vi "TSM SSC DCPower Finish Waveform Acquisition.vi"(0 "DCPower SSC in":T3, 1 "Settings":T1 {"Previous Settings"."Triggers:Measure Trigger:Trigger Type" items=["Digital Edge"=1014, "Software Edge"=1015, "None"=1012]; "Previous Settings"."Measurement:Advanced:Measure When" items=["Automatically after Source Complete"=1025, "On Demand"=1026, "On Measure Trigger"=1027]; "Previous Settings"."Measurement:Aperture Time" format="%#_6p"; "Previous Settings"."Measurement:Aperture Time Units" items=["Seconds"=1028, "Power Line Cycles"=1029]}, 5 "Fetch Waveform Length (s)":dbl, 11 "error in":errorcluster) -> (4 "DCPower SSC out":T3, 6 "Voltage Waveforms":waveform(dbl)[](graph), 8 "Current Waveforms":waveform(dbl)[](graph), 15 "error out":errorcluster)   [LabVIEW 2019]
doc: "This VI reconfigures the SMU to the previous settings and outputs the samples captured during waveform acquisition."
uses:
  TSM/TSM SSC DCPower.ctl
  <vilib>/NI_TestStand_SemiconductorModule/NI_TestStand_Semiconductor_Module.lvlibp/PinMap/PinQueryContext/MultiplePinMultipleSessionQueryContext/MultiplePinMultipleSessionQueryContext.lvclass
  SSC DCPower/SSC DCPower.ctl
  Shared SubVIs/TSM Pin Abstraction/TSM Pin Information.ctl
  Shared SubVIs/TSM Pin Abstraction/TSM Pin Type Identifier.ctl
  Shared SubVIs/TSM Pin Abstraction/TSM Expanded Pin Information.ctl
  SSC DCPower/Waveform Acquisition/SSC DCPower Waveform Acquisition Saved Settings.ctl
  SSC DCPower/Waveform Acquisition/SSC DCPower Waveform Acquisition Saved Setting.ctl
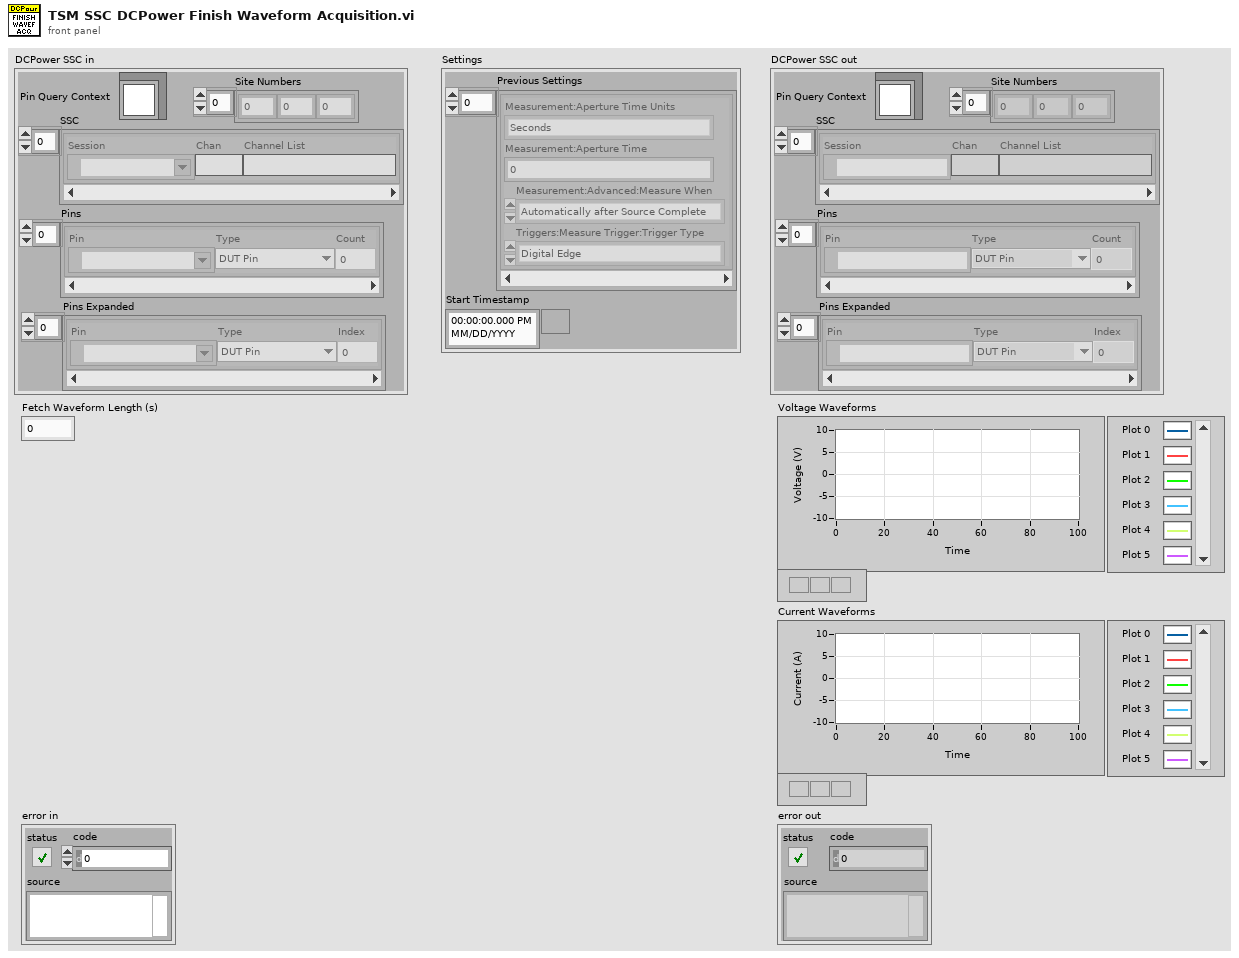
[diagram p1: front panel]
types:
  T1 = typedef "SSC DCPower Waveform Acquisition Saved Settings.ctl" = cluster{"Previous Settings":T2[], "Start Timestamp":timestamp}
  T2 = typedef "SSC DCPower Waveform Acquisition Saved Setting.ctl" = cluster{"Measurement:Aperture Time Units":i32, "Measurement:Aperture Time":dbl, "Measurement:Advanced:Measure When":i32, "Triggers:Measure Trigger:Trigger Type":i32}
  T3 = typedef "TSM SSC DCPower.ctl" = cluster{"Pin Query Context":refnum<class "MultiplePinMultipleSessionQueryContext.lvclass">, "SSC":T4[], "Site Numbers":i32[], "Pins":T5[], "Pins Expanded":T7[]}
  T4 = typedef "SSC DCPower.ctl" = cluster{"Session":refnum<k15>, "Chan":string, "Channel List":string}
  T5 = typedef "TSM Pin Information.ctl" = cluster{"Pin":tag, "Type":T6, "Count":i32}
  T6 = typedef "TSM Pin Type Identifier.ctl" = enum8{"DUT Pin", "System Pin", "Pin Group", "Not Determined"}
  T7 = typedef "TSM Expanded Pin Information.ctl" = cluster{"Pin":tag, "Type":T6, "Index":i32}
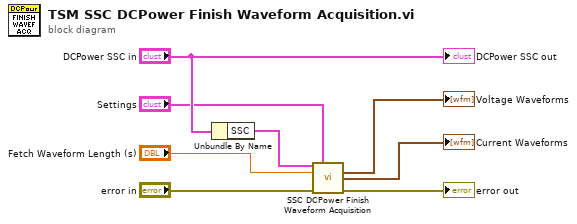
[diagram p0: block diagram]
diagram:
  n1 = Unbundle By Name("DCPower SSC in") -> ("SSC"=w5:T4[])
  n2 = call "SSC DCPower Finish Waveform Acquisition.vi"("DCPower SSC in"=w5, "Settings"="Settings", "Fetch Waveform Length (s)"="Fetch Waveform Length (s)", "error in"="error in") -> ("Voltage Waveforms"=→"Voltage Waveforms":waveform(dbl)[], "Current Waveforms"=→"Current Waveforms":waveform(dbl)[], "error out"=→"error out":errorcluster)  [unwired: 8 in, 1 out]
  "DCPower SSC out" <- "DCPower SSC in"
